vi "GUI_laptop v4.vi"() -> ()   [LabVIEW 2019]
uses:
  <vilib>/Math Plots/3D Math Plots/3D Scatter/3D Scatter XCtrl/3D Scatter.xctl
  <vilib>/Platform/TimedLoop/XDataNode/timing_clust.ctl
  <vilib>/Platform/TimedLoop/XDataNode/nitl_modes.ctl
  <vilib>/Platform/TimedLoop/XDataNode/wakeup.ctl
  <vilib>/Analysis/_algsub.llb/Real Vector Norm.vi
  <vilib>/Instr/_visa.llb/VISA Configure Serial Port (Instr).vi
  <vilib>/Math Plots/3D Math Plots/3D Scatter/3D Scatter Datatype/Public/Plot Helper (Vector).vi
  <vilib>/Utility/file.llb/Write Delimited Spreadsheet (DBL).vi
  <vilib>/platform/TimedLoop/XDataNode/XDataNode.xnode
  <vilib>/Platform/TimedLoop/XDataNode/XDNodeRunTimeDep.lvlib
  <vilib>/Math Plots/3D Math Plots/3D Scatter/3D Scatter Datatype/3D Scatter Datatype.lvclass
  <vilib>/Analysis/NI_AALPro.lvlib
panel:
  out "Numeric":i32
  in  "L5 bound":dbl=0.5
  in  "L4 bound (deg)":dbl=0.5
  in  "L3 bound (mm)":dbl=0.5
  in  "L2 bound (deg)":dbl=0.5
  in  "L1 bound (deg)":dbl=0.5
  in  "Joystick Type":dbl(ring) items=["Rigid Joystick", "Free Joystick"]
  out "Finished Late? [i-1]":bool
  in  "Epsilon":dbl=0.2
  out "3D Scatter":refnum<class "3D Plot Datatype.lvclass">[](xcontrol)
  out "Random Point":dbl[](array[numeric])
  out "Virtual Cursor":dbl[](array[numeric])
  out "Iteration Duration":i64
  in  "Num of Points":i32=10
  in  "z bound":dbl=2.0
  in  "y bound":dbl=5.0
  in  "x bound":dbl=5.0
  in  "Stop":bool
  in  "Round Decimals":dbl=2.0 format="%#_15g"
  in  "Save  Data":bool
  in  "Save Path":path
  in  "x speed":dbl=0.5
  in  "z speed":dbl=0.5
  in  "y speed":dbl=0.5
  out "error out":errorcluster
  in  "baud rate":u32=115200
  in  "VISA resource name":refnum<visa-resource-name>
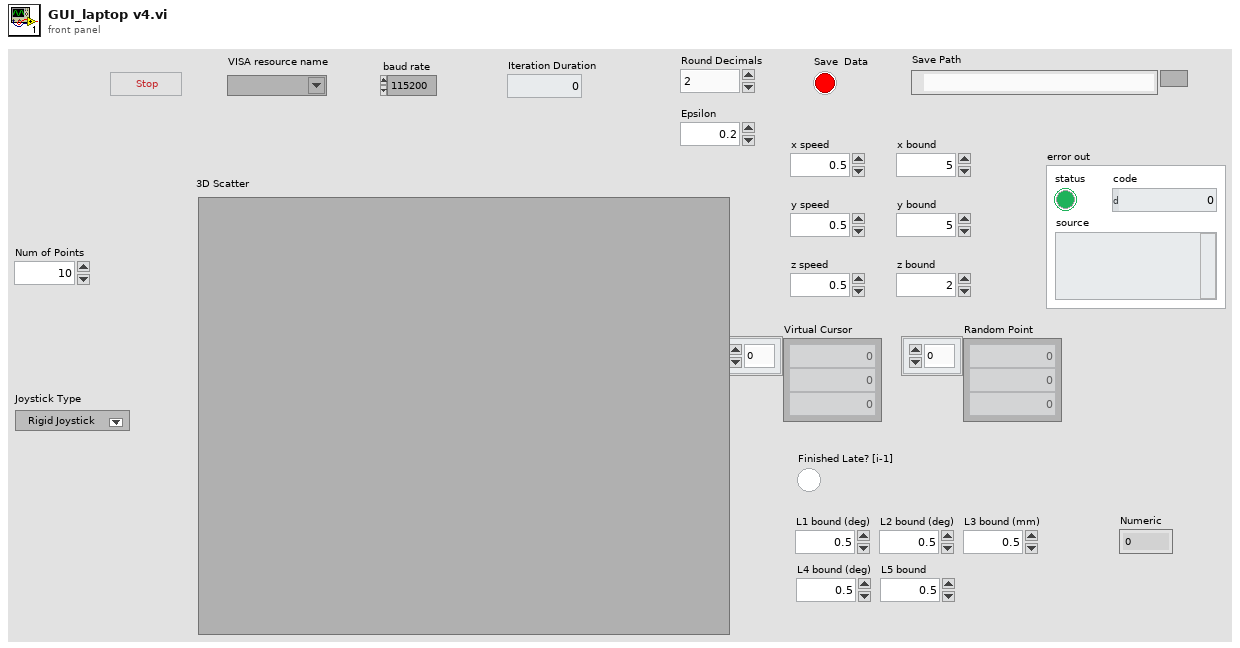
[diagram p1: front panel]
types:
  T1 = typedef "XDNodeRunTimeDep.lvlib/timing_clust.ctl" = cluster{"Expected End [f-1]":u64, "Actual End [f-1]":u64, "Finished Late? [f-1]":bool, "Expected End [i-1]":u64, "Actual End [i-1]":u64, "Finished Late? [i-1]":bool, "Expected Start [i]":u64, "Actual Start [i]":u64, "Expected Start [f]":u64, "Actual Start [f]":u64, "Source Name":string, "Structure Name":string, "Period":i64, "Deadline":i64, "Offset":i64, "Start":i64, "Priority":i32, "Timeout":i32, "Mode":T2, "Wakeup Reason":T3, "Error":errorcluster, "Source Type":string, "Secondary Source Type":string, "Global End Time":u64, "Global Start Time":u64, "Frame Duration":u64, "Iteration Duration":u64, "Assigned CPU":i32, "I/O Scan Engine Mode":u32}
  T2 = typedef "XDNodeRunTimeDep.lvlib/nitl_modes.ctl" = enum32{"No Change", "Process missed periods, maintain original phase", "Discard missed periods, maintain original phase", "Process missed periods, ignore original phase", "Discard missed periods, ignore original phase"}
  T3 = typedef "XDNodeRunTimeDep.lvlib/wakeup.ctl" = enum32{"Normal", "Aborted", "Asynchronous wakeup", "Timing source error", "Timed loop error", "Timeout"}
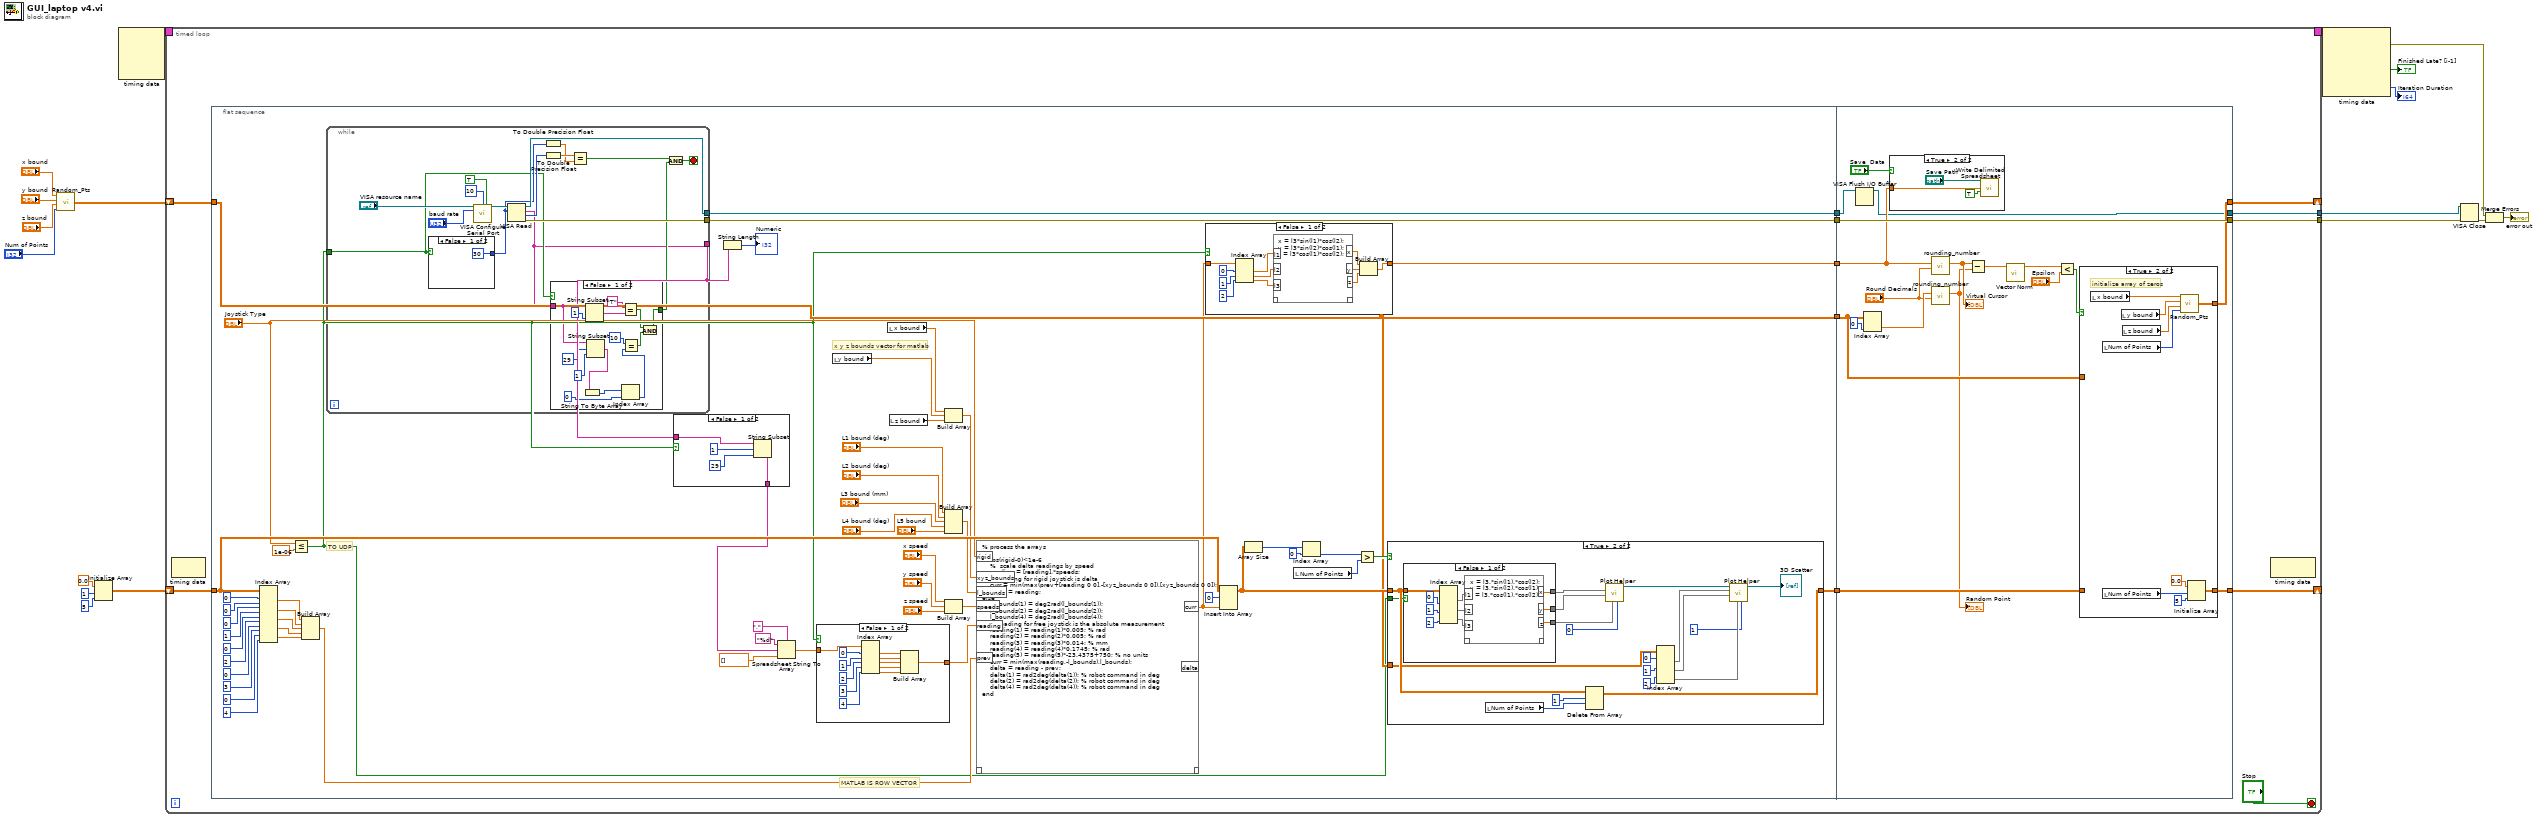
[diagram p0: block diagram]
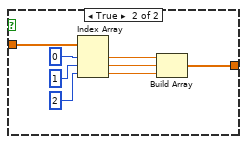
[diagram p3: hidden frame]
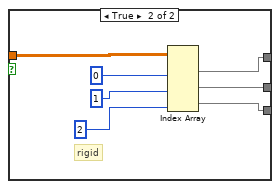
[diagram p6: hidden frame]
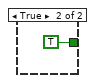
[diagram p7: hidden frame]
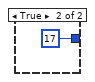
[diagram p8: hidden frame]
diagram:
  n1 = call "Random_Pts.vi"("Num of Points"="Num of Points", "z bound"="z bound", "y bound"="y bound", "x bound"="x bound") -> ("appended array"=w4:dbl[][])
  n2 = Initialize Array(0.0 ("element"), 1 ("dimension size"), 5 ("dimension size")) -> (w11:dbl[][])
  n3 = node-c288() -> (w18:T1)  [unwired: 4 in]
  n4 = timed-loop {
    tunnel: [w29] -> w13
    tunnel: [w28] -> w12
    shift-right: [w27] -> _
    shift-left: w11 -> [w26]
    timing: w18 -> [_]
    timing-out: [_] -> w17
    shift-right: [w19] -> _
    shift-left: w4 -> [w21]
    stop <- "Stop" stop-if-true
    n5 = node-c288() -> ()  [unwired: 1 in, 1 out]
    n6 = flat-sequence {
      tunnel: w26 -> [w73]
      tunnel: [w68] -> w25
      tunnel: [w85] -> w24
      tunnel: [w69] -> w23
      tunnel: [w47] -> w22
      tunnel: w21 -> [w67]
      tunnel: [w67] -> w20
      tunnel: w25 -> [w196]
      tunnel: w24 -> [w212]
      tunnel: w23 -> [w205]
      tunnel: w22 -> [w207]
      tunnel: w20 -> [w209]
      tunnel: [w195] -> w29
      tunnel: [w212] -> w28
      tunnel: [w204] -> w27
      tunnel: [w208] -> w19
      frame #0 {
        # "TO UDP"
        # "MATLAB IS ROW VECTOR"
        # "x y z bounds vector for matlab"
        n7 = Index Array(array=w73, index (row) #1=0 ("disabled index (row)"), index (col) #1=0 ("disabled index (col)"), index (row) #2=0 ("disabled index (row)"), index (col) #2=1 ("disabled index (col)"), index (row) #3=0 ("disabled index (row)"), index (col) #3=2 ("disabled index (col)"), index (row) #4=0 ("disabled index (row)"), index (col) #4=3 ("disabled index (col)"), index (row) #5=0 ("disabled index (row)"), index (col) #5=4 ("disabled index (col)")) -> (element #1=w60:dbl, element #2=w59:dbl, element #3=w58:dbl, element #4=w42:dbl, element #5=w41:dbl)
        n8 = Less Or Equal?(x="Joystick Type", y=1e-06) -> (x <= y?=w34:bool)
        n9 = Build Array(w60, w59, w58, w42, w41) -> (w57:dbl[])
        n10 = while {
          tunnel: [w162] -> w35
          tunnel: [w175] -> w85
          tunnel: [w169] -> w68
          tunnel: w34 -> [w163]
          stop <- w165 stop-if-true
          n11 = case shown="False" w163 {
            tunnel: [30 u32 17 ("byte count")] -> w168
            frame False {
            }
            frame True {
            }
          }
          n12 = call-poly "VISA Configure Serial Port"("VISA resource name"="VISA resource name", "termination char\n(0xA = '\\n' = LF)"=u8 10 ("termination char\n(0xA = '\\n' = LF)"), "Enable Termination\nChar (T)"=TRUE ("Enable Termination\nChar (T)"), "baud rate (9600)"="baud rate") -> ("VISA resource name out"=w170:refnum<visa-resource-name>)  [unwired: 10 in, 1 out]
          n13 = VISA Read(VISA resource name=w170, byte count=w168) -> (VISA resource name out=w169:refnum<visa-resource-name>, read buffer=w162:string, return count=w177:u32, error out=w175:errorcluster)  [unwired: 1 in]
          n14 = To Double Precision Float(number=w168) -> (double precision float=w167:dbl)
          n15 = To Double Precision Float(number=w177) -> (double precision float=w176:dbl)
          n16 = case shown="False" w163 {
            tunnel: [w184 TRUE] -> w164
            tunnel: w162 -> [w187 _]
            frame False {
              n17 = String Subset(string=w187, length (rest)=1) -> (substring=w190:string)  [unwired: 1 in]
              n18 = String Subset(string=w187, offset (0)=29, length (rest)=1) -> (substring=w182:string)
              n19 = String To Byte Array(string=w182) -> (unsigned byte array=w181:u8[])
              n20 = Equal?(x="T", y=w190) -> (x = y?=w186:bool)
              n21 = Index Array(array=w181, index=0) -> (element=w179:u8)
              n22 = Equal?(x=10, y=w179) -> (x = y?=w185:bool)
              n23 = And(x=w186, y=w185) -> (x .and. y?=w184:bool)
            }
            frame True {
            }
          }
          n24 = Equal?(x=w176, y=w167) -> (x = y?=w166:bool)
          n25 = And(x=w166, y=w164) -> (x .and. y?=w165:bool)
        }
        n26 = case shown="False" w34 {
          tunnel: w35 -> [w91 w92]
          tunnel: [w88 w92] -> w33
          frame False {
            n27 = String Subset(string=w91, offset (0)=1, length (rest)=29) -> (substring=w88:string)
          }
          frame True {
          }
        }
        n28 = String Length(string=w35) -> (length=→"Numeric":i32)
        n29 = Spreadsheet String To Array(delimiter (Tab)=",", format string="%d", spreadsheet string=w33, array type (2D Dbl)=dbl[] []) -> (array=w38:dbl[])
        n30 = case shown="False" w34 {
          tunnel: w38 -> [w93 w106]
          tunnel: [w98 w105] -> w37
          frame False {
            n31 = Index Array(array=w93, index #1=0 ("Plot ID"), index #2=1 ("Plot ID"), index #3=2 ("Plot ID"), index #4=3 ("Plot ID"), index #5=4 ("Plot ID")) -> (element #1=w101:dbl, element #2=w100:dbl, element #3=w99:dbl, element #4=w95:dbl, element #5=w94:dbl)
            n32 = Build Array(w101, w100, w99, w95, w94) -> (w98:dbl[])
          }
          frame True {
            n33 = Index Array(array=w106, index #1=0 ("Plot ID"), index #2=1 ("Plot ID"), index #3=2 ("Plot ID")) -> (element #1=w109:dbl, element #2=w108:dbl, element #3=w107:dbl)
            n34 = Build Array(w109, w108, w107) -> (w105:dbl[])
          }
        }
        n35 = local read "y bound"() -> (w62:dbl)
        n36 = local read "x bound"() -> (w63:dbl)
        n37 = local read "z bound"() -> (w61:dbl)
        n38 = Build Array(w63, w62, w61) -> (w55:dbl[])
        n39 = Build Array("L1 bound (deg)", "L2 bound (deg)", "L3 bound (mm)", "L4 bound (deg)", "L5 bound") -> (w51:dbl[])
        n40 = Build Array("x speed", "y speed", "z speed") -> (w56:dbl[])
        n41 = script code="% process the arrays\n\nif abs(rigid-0)<1e-6\n    %  scale delta readings by speed\n    reading = [reading].*speeds;\n    % reading for rigid joystick is delta\n    curr = min(max(prev+[reading 0 0],-[xyz_bounds 0 0]),[xyz_bounds 0 0]);\n    delta = reading;\nelse\n    l_bounds(1) = deg2rad(l_bounds(1));\n    l_bounds(2) = deg2rad(l_bounds(2));\n    l_bounds(4) = deg2rad(l_bounds(4));\n    % reading for free joystick is the absolute measurement\n    reading(1) = reading(1)*0.005; % rad\n    reading(2) = reading(2)*0.005; % rad\n    reading(3) = reading(3)*0.014; % mm\n    reading(4) = reading(4)*0.1745; % rad\n    reading(5) = reading(5)*-23.4375+750; % no units\n    curr = min(max(reading,-l_bounds),l_bounds);\n    delta = reading - prev;\n    delta(1) = rad2deg(delta(1)); % robot command in deg\n    delta(2) = rad2deg(delta(2)); % robot command in deg\n    delta(4) = rad2deg(delta(4)); % robot command in deg\nend"("xyz_bounds"=w55, "speeds"=w56, "reading"=w37, "prev"=w57, "rigid"="Joystick Type", "l_bounds"=w51) -> ("curr"=w48:dbl[])  [unwired: 1 in, 2 out]
        n42 = case shown="False" w34 {
          tunnel: w48 -> [w120 w124]
          tunnel: [w113 w124] -> w47
          frame False {
            n43 = Index Array(array=w120, index #1=0 ("Plot ID"), index #2=1 ("Plot ID"), index #3=2 ("Plot ID")) -> (element #1=w119:dbl, element #2=w118:dbl, element #3=w117:dbl)
            n44 = script code="x = l3*sin(l1)*cos(l2);\ny = l3*sin(l2)*cos(l1);\nz = l3*cos(l1)*cos(l2);"("l1"=w119, "l2"=w118, "l3"=w117) -> ("x"=w116:dbl, "y"=w115:dbl, "z"=w114:dbl)  [unwired: 1 in, 1 out]
            n45 = Build Array(w116, w115, w114) -> (w113:dbl[])
          }
          frame True {
          }
        }
        n46 = Insert Into Array(array=w73, index (row)=0, new element=w48) -> (w71:dbl[][])  [unwired: 1 in]
        n47 = Array Size(array=w71) -> (size(s)=w74:i32[])
        n48 = local read "Num of Points"() -> (w72:i32)
        n49 = Index Array(array=w74, index=0) -> (element=w75:i32)
        n50 = Greater?(x=w75, y=w72) -> (0:w70:bool)
        n51 = case shown="True" w70 {
          tunnel: w71 -> [w125 w143]
          tunnel: [w125 w142] -> w69
          tunnel: w67 -> [_ w141]
          tunnel: w34 -> [_ w126]
          frame False {
          }
          frame True {
            n52 = case shown="False" w126 {
              tunnel: w143 -> [w154 w158]
              tunnel: [w145 w157] -> w132
              tunnel: [w146 w156] -> w131
              tunnel: [w147 w155] -> w130
              frame False {
                n53 = Index Array(array=w154, index (col) #1=0 ("Plot ID"), index (col) #2=1 ("Plot ID"), index (col) #3=2 ("Plot ID")) -> (element #1=w150:dbl[], element #2=w149:dbl[], element #3=w148:dbl[])  [unwired: 3 in]
                n54 = script code="x = l3.*sin(l1).*cos(l2);\ny = l3.*sin(l2).*cos(l1);\nz = l3.*cos(l1).*cos(l2);"("l1"=w150, "l2"=w149, "l3"=w148) -> ("x"=w145:dbl[], "y"=w146:dbl[], "z"=w147:dbl[])  [unwired: 1 in, 1 out]
              }
              frame True {
                # "rigid"
                n55 = Index Array(array=w158, index (col) #1=0 ("disabled index (col)"), index (col) #2=1 ("index (col)"), index (col) #3=2 ("index (col)")) -> (element #1=w157:dbl[], element #2=w156:dbl[], element #3=w155:dbl[])  [unwired: 3 in]
              }
            }
            n56 = local read "Num of Points"() -> (w140:i32)
            n57 = Delete From Array(array=w143, length=1, index (row)=w140) -> (array with subset deleted=w142:dbl[][])  [unwired: 1 in, 1 out]
            n58 = call-poly <vilib>:"Plot Helper.vi"("Plot ID"=0, "z vector"=w130, "y vector"=w131, "x vector"=w132) -> ("3D Plot lvclass Array out"=w134:refnum<class "3D Plot Datatype.lvclass">[])  [unwired: 2 in, 5 out]
            n59 = Index Array(array=w141, index (row) #1=0 ("index (row)"), index (row) #2=1 ("index (row)"), index (row) #3=2 ("index (row)")) -> (element #1=w138:dbl[], element #2=w137:dbl[], element #3=w136:dbl[])  [unwired: 3 in]
            n60 = call-poly <vilib>:"Plot Helper.vi"("Plot ID"=1, "z vector"=w136, "y vector"=w137, "x vector"=w138, "3D Plot lvclass Array in"=w134) -> ("3D Plot lvclass Array out"=→"3D Scatter":refnum<class "3D Plot Datatype.lvclass">[])  [unwired: 1 in, 5 out]
          }
        }
      }
      frame #1 {
        n61 = VISA Flush I/O Buffer(VISA resource name=w196) -> (VISA resource name out=w195:refnum<visa-resource-name>)  [unwired: 2 in, 1 out]
        n62 = Index Array(array=w209, index (col)=0 ("index (row)")) -> (element=w211:dbl[])  [unwired: 1 in]
        n63 = case shown="True" "Save  Data" {
          tunnel: w207 -> [_ w213]
          frame False {
          }
          frame True {
            n64 = call-poly <vilib>:"Write Delimited Spreadsheet.vi"("file path (dialog if empty)"="Save Path", "1D data"=w213, "append to file? (new file:F)"=TRUE) -> ()  [unwired: 11 in, 2 out]
          }
        }
        n65 = call "rounding_number.vi"("power of ten"="Round Decimals", "Array"=w207) -> ("rounded"=w203:dbl[])  [unwired: 9 in]
        "Virtual Cursor" <- w203
        n66 = call "rounding_number.vi"("power of ten"="Round Decimals", "Array"=w211) -> ("rounded"=w202:dbl[])  [unwired: 9 in]
        "Random Point" <- w202
        n67 = Subtract(x=w203, y=w202) -> (x-y=w201:dbl[])
        n68 = call-poly <vilib>:"Vector Norm.vi"("Input Vector"=w201) -> ("norm"=w200:dbl)  [unwired: 9 in, 1 out]
        n69 = Less?(x=w200, y="Epsilon") -> (x < y?=w198:bool)
        n70 = case shown="True" w198 {
          tunnel: w209 -> [w217 _]
          tunnel: [w217 w222] -> w208
          tunnel: w205 -> [w216 _]
          tunnel: [w216 w218] -> w204
          frame False {
          }
          frame True {
            # "initialize array of zeros"
            n71 = local read "x bound"() -> (w226:dbl)
            n72 = local read "Num of Points"() -> (w223:i32)
            n73 = local read "Num of Points"() -> (w220:i32)
            n74 = local read "y bound"() -> (w225:dbl)
            n75 = local read "z bound"() -> (w224:dbl)
            n76 = call "Random_Pts.vi"("Num of Points"=w223, "z bound"=w224, "y bound"=w225, "x bound"=w226) -> ("appended array"=w222:dbl[][])
            n77 = Initialize Array(0.0 ("element"), w220, 5 ("dimension size")) -> (w218:dbl[][])
          }
        }
      }
    }
    n78 = node-c288() -> ()  [unwired: 1 in, 1 out]
  }
  n79 = node-c288(w17) -> (w10:errorcluster, →"Finished Late? [i-1]":bool, →"Iteration Duration":i64)  [unwired: 3 out]
  n80 = VISA Close(VISA resource name=w13, error in (no error)=w12) -> (error out=w9:errorcluster)
  n81 = Merge Errors(w10, w9) -> (→"error out":errorcluster)
